vi "Node Type.vi"(4 "Parser State":T2) -> (6 "Next":i32, 7 "Value Type":T1)   [LabVIEW 2020, in "CDM-Config.lvlib" / "Config-YAML.lvclass"]
uses:
  Config-YAML.lvclass
  Config-YAML.lvclass/Config-YAML.ctl
  Value Type.ctl
  CDM-Config.lvlib
  Parser State.ctl
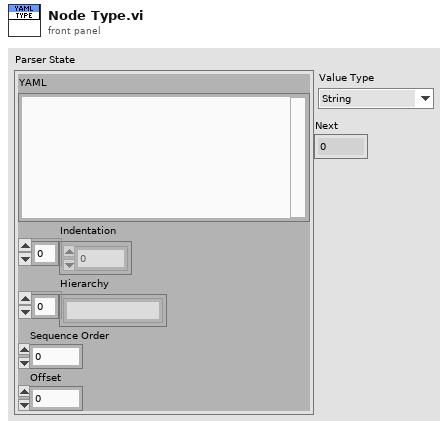
[diagram p1: front panel]
types:
  T1 = typedef "CDM-Config.lvlib/Value Type.ctl" = enum16{"String", "Number", "Bool", "Object", "Array"}
  T2 = typedef "CDM-Config.lvlib/Config-YAML.lvclass/Parser State.ctl" = cluster{"YAML":string, "Indentation":i32[], "Hierarchy":string[], "Sequence Order":i32, "Offset":i32}
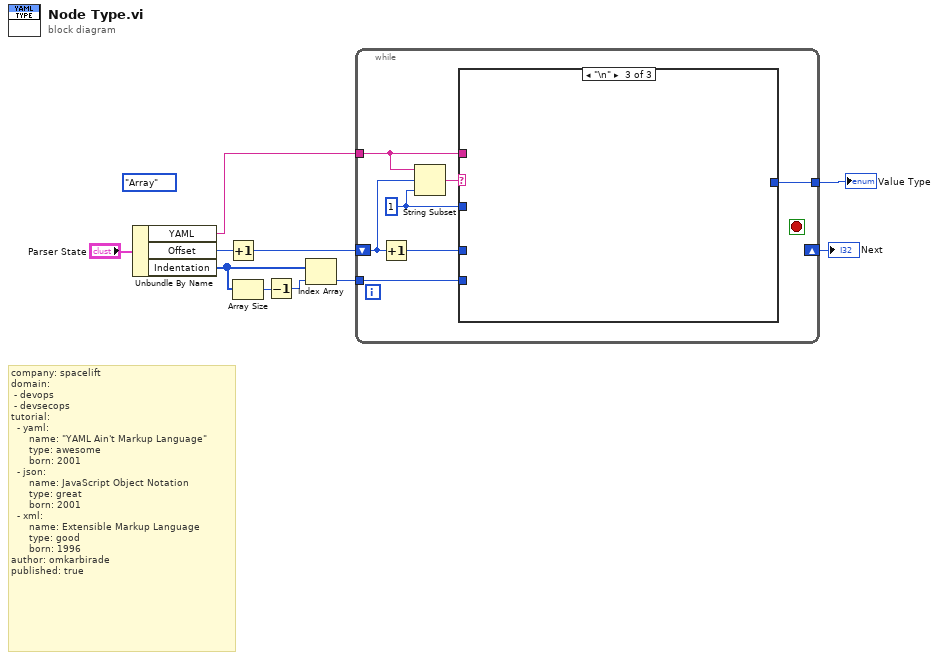
[diagram p0: block diagram]
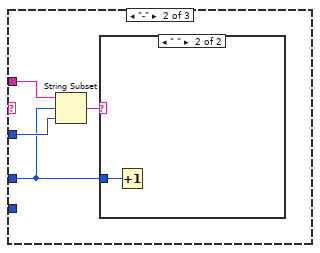
[diagram p3: hidden frame]
diagram:
  (unwired) Value_Type."Array" ("Value Type")
  # "company: spacelift\ndomain:\n - devops\n - devsecops\ntutorial:\n  - yaml:\n      name: \"YAML Ain't Markup Language\"\n      type: awesome\n      born: 2001\n  - json:\n      name: JavaScript Object Notation\n      type: great\n      born: 2001\n  - xml:\n      name: Extensible Markup Language\n      type: good\n      born: 1996\nauthor: omkarbirade\npublished: true"
  n1 = Unbundle By Name("Parser State") -> ("YAML"=w8:string, "Offset"=w9:i32, "Indentation"=w3:i32[])
  n2 = Increment(x=w9) -> (x+1=w6:i32)
  n3 = Array Size(array=w3) -> (size(s)=w4:i32)
  n4 = Decrement(x=w4) -> (x-1=w2:i32)
  n5 = Index Array(array=w3, index=w2) -> (element=w1:i32)
  n6 = while {
    shift-right: [_] -> w5
    shift-left: w6 -> [w16]
    tunnel: w8 -> [w12]
    tunnel: [w15] -> w7
    tunnel: w1 -> [w11]
    stop <- _ stop-if-true
    w13 = 1 ("length (rest)")
    n7 = Increment(x=w16) -> (x+1=w14:i32)
    n8 = String Subset(string=w12, offset (0)=w16, length (rest)=w13) -> (substring=w17:string)
    n9 = case shown="\"\\n\"" w17 {
      tunnel: [_ _ _] -> w15
      tunnel: w14 -> [_ w18 _]
      tunnel: w13 -> [_ w21 _]
      tunnel: w12 -> [_ w20 _]
      tunnel: w11 -> [_ _ _]
      frame Default {
      }
      frame "-" {
        n10 = String Subset(string=w20, offset (0)=w18, length (rest)=w21) -> (substring=w19:string)
        n11 = case shown="\" \"" w19 {
          tunnel: w18 -> [_ w22]
          frame Default {
          }
          frame " " {
            n12 = Increment(x=w22) -> ()  [unwired: 1 out]
          }
        }
      }
      frame "\n" {
      }
    }
  }
  "Value Type" <- w7
  "Next" <- w5
